vi "Strip Path Extension Path.vi"(0 "path":path) -> (1 "root":string, 2 "extension":string)   [LabVIEW 2012, in "Path Function.lvlib"]
uses:
  Path Function.lvlib
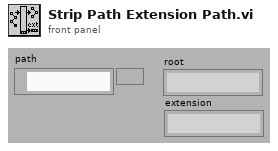
[diagram p1: front panel]
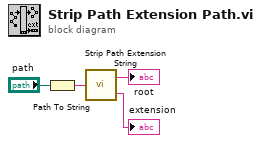
[diagram p0: block diagram]
diagram:
  n1 = Path To String(path="path") -> (string=w3:string)
  n2 = call "Strip Path Extension String.vi"("path"=w3) -> ("root"=→"root":string, "extension"=→"extension":string)
